vi "test_libssh2_sftp_close_handle.vi"() -> ()   [LabVIEW 2017, in "integration_tests.lvlib"]
uses:
  integration_tests.lvlib
  support/support.lvlib
  libssh2/libssh2.lvlib
  <vilib>/PNR/Transparent Assertions/Transparent Assertions/Transparent Assertions.lvlib
panel:
  out "error out":errorcluster
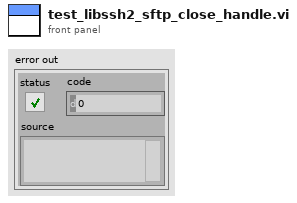
[diagram p1: front panel]
types:
  T1 = typedef "libssh2.lvlib/Session Refnum.ctl" = refnum<k1>
  T2 = typedef "libssh2.lvlib/SFTP Refnum.ctl" = refnum<k1>
  T3 = typedef "libssh2.lvlib/SFTP Handle Refnum.ctl" = refnum<k1>
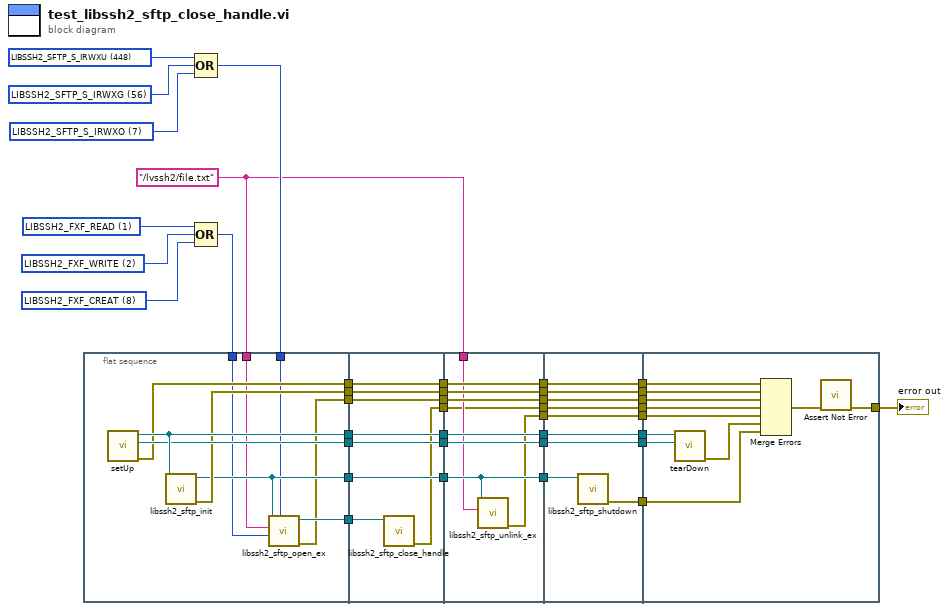
[diagram p0: block diagram]
diagram:
  w34 = u32 2 items=["LIBSSH2_FXF_READ"=1, "LIBSSH2_FXF_WRITE"=2, "LIBSSH2_FXF_APPEND"=4, "LIBSSH2_FXF_CREAT"=8, "LIBSSH2_FXF_TRUNC"=16, "LIBSSH2_FXF_EXCL"=32] ("flags")
  w35 = u32 1 items=["LIBSSH2_FXF_READ"=1, "LIBSSH2_FXF_WRITE"=2, "LIBSSH2_FXF_APPEND"=4, "LIBSSH2_FXF_CREAT"=8, "LIBSSH2_FXF_TRUNC"=16, "LIBSSH2_FXF_EXCL"=32] ("flags")
  w33 = u32 8 items=["LIBSSH2_FXF_READ"=1, "LIBSSH2_FXF_WRITE"=2, "LIBSSH2_FXF_APPEND"=4, "LIBSSH2_FXF_CREAT"=8, "LIBSSH2_FXF_TRUNC"=16, "LIBSSH2_FXF_EXCL"=32] ("flags")
  w4 = "/lvssh2/file.txt" ("filename")
  w37 = 7 items=["LIBSSH2_SFTP_S_IRWXU"=448, "LIBSSH2_SFTP_S_IRUSR"=256, "LIBSSH2_SFTP_S_IWUSR"=128, "LIBSSH2_SFTP_S_IXUSR"=64, "LIBSSH2_SFTP_S_IRWXG"=56, "LIBSSH2_SFTP_S_IRGRP"=32, "LIBSSH2_SFTP_S_IWGRP"=16, "LIBSSH2_SFTP_S_IXGRP"=8, "LIBSSH2_SFTP_S_IRWXO"=7, "LIBSSH2_SFTP_S_IROTH"=4, "LIBSSH2_SFTP_S_IWOTH"=2, "LIBSSH2_SFTP_S_IXOTH"=1] ("mode")
  w38 = 56 items=["LIBSSH2_SFTP_S_IRWXU"=448, "LIBSSH2_SFTP_S_IRUSR"=256, "LIBSSH2_SFTP_S_IWUSR"=128, "LIBSSH2_SFTP_S_IXUSR"=64, "LIBSSH2_SFTP_S_IRWXG"=56, "LIBSSH2_SFTP_S_IRGRP"=32, "LIBSSH2_SFTP_S_IWGRP"=16, "LIBSSH2_SFTP_S_IXGRP"=8, "LIBSSH2_SFTP_S_IRWXO"=7, "LIBSSH2_SFTP_S_IROTH"=4, "LIBSSH2_SFTP_S_IWOTH"=2, "LIBSSH2_SFTP_S_IXOTH"=1] ("mode")
  w39 = 448 items=["LIBSSH2_SFTP_S_IRWXU"=448, "LIBSSH2_SFTP_S_IRUSR"=256, "LIBSSH2_SFTP_S_IWUSR"=128, "LIBSSH2_SFTP_S_IXUSR"=64, "LIBSSH2_SFTP_S_IRWXG"=56, "LIBSSH2_SFTP_S_IRGRP"=32, "LIBSSH2_SFTP_S_IWGRP"=16, "LIBSSH2_SFTP_S_IXGRP"=8, "LIBSSH2_SFTP_S_IRWXO"=7, "LIBSSH2_SFTP_S_IROTH"=4, "LIBSSH2_SFTP_S_IWOTH"=2, "LIBSSH2_SFTP_S_IXOTH"=1] ("mode")
  n1 = flat-sequence {
    tunnel: [w50] -> w26
    tunnel: [w49] -> w25
    tunnel: [w46] -> w24
    tunnel: [w48] -> w23
    tunnel: [w47] -> w22
    tunnel: w36 -> [w45]
    tunnel: w4 -> [w44]
    tunnel: w32 -> [w43]
    tunnel: [w42] -> w21
    tunnel: [w41] -> w20
    tunnel: w26 -> [w58]
    tunnel: [w58] -> w18
    tunnel: w25 -> [w57]
    tunnel: [w57] -> w16
    tunnel: w24 -> [w56]
    tunnel: [w56] -> w14
    tunnel: w23 -> [w55]
    tunnel: [w55] -> w12
    tunnel: w22 -> [w54]
    tunnel: [w54] -> w10
    tunnel: w21 -> [w53]
    tunnel: w20 -> [w52]
    tunnel: [w52] -> w8
    tunnel: [w51] -> w3
    tunnel: w18 -> [w67]
    tunnel: [w67] -> w17
    tunnel: w16 -> [w66]
    tunnel: [w66] -> w15
    tunnel: w14 -> [w62]
    tunnel: [w62] -> w13
    tunnel: w12 -> [w65]
    tunnel: [w65] -> w11
    tunnel: w10 -> [w64]
    tunnel: [w64] -> w9
    tunnel: w8 -> [w63]
    tunnel: [w63] -> w7
    tunnel: [w61] -> w5
    tunnel: w4 -> [w60]
    tunnel: w3 -> [w59]
    tunnel: [w59] -> w2
    tunnel: w17 -> [w76]
    tunnel: [w76] -> w31
    tunnel: w15 -> [w75]
    tunnel: [w75] -> w30
    tunnel: w13 -> [w72]
    tunnel: w11 -> [w74]
    tunnel: [w74] -> w29
    tunnel: w9 -> [w73]
    tunnel: [w73] -> w28
    tunnel: [w71] -> w27
    tunnel: w7 -> [w70]
    tunnel: [w70] -> w19
    tunnel: [w69] -> w6
    tunnel: w5 -> [w69]
    tunnel: w2 -> [w68]
    tunnel: [w68] -> w1
    tunnel: w31 -> [w87]
    tunnel: w30 -> [w86]
    tunnel: w29 -> [w85]
    tunnel: [w82] -> w40
    tunnel: w28 -> [w81]
    tunnel: w27 -> [w80]
    tunnel: w19 -> [w79]
    tunnel: w6 -> [w78]
    tunnel: w1 -> [w77]
    frame #0 {
      n2 = call "setUp.vi"() -> ("error out"=w48:errorcluster, "connection ID"=w49:refnum<k5>, "session"=w50:T1)  [unwired: 9 in]
      n3 = call "libssh2_sftp_init.vi"("session"=w50) -> ("error out"=w47:errorcluster, "sftp"=w46:T2)  [unwired: 9 in]
      n4 = call "libssh2_sftp_open_ex.vi"("mode"=w45, "flags"=w43, "filename"=w44, "sftp"=w46) -> ("error out"=w41:errorcluster, "sftp handle"=w42:T3)  [unwired: 6 in]
    }
    frame #1 {
      n5 = call "libssh2_sftp_close_handle.vi"("sftp handle"=w53) -> ("error out"=w51:errorcluster)  [unwired: 10 in]
    }
    frame #2 {
      n6 = call "libssh2_sftp_unlink_ex.vi"("file"=w60, "sftp"=w62) -> ("error out"=w61:errorcluster)  [unwired: 9 in]
    }
    frame #3 {
      n7 = call "libssh2_sftp_shutdown.vi"("sftp"=w72) -> ("error out"=w71:errorcluster)  [unwired: 10 in]
    }
    frame #4 {
      n8 = call "tearDown.vi"("connection ID"=w86, "session"=w87) -> ("error out"=w84:errorcluster)  [unwired: 9 in]
      n9 = Merge Errors(w85, w81, w79, w77, w78, w84, w80) -> (w83:errorcluster)
      n10 = call <vilib>:"Assert Not Error.vi"("error in (no error)"=w83) -> ("error out"=w82:errorcluster)  [unwired: 10 in]
    }
  }
  n11 = Compound Arithmetic op=OR(w39, w38, w37) -> (w36:i32)
  n12 = Compound Arithmetic op=OR(w35, w34, w33) -> (w32:u32)
  "error out" <- w40
